vi "JSON to Array of Cluster.vi"(5 "JSON":string, 6 "JSONtext LVClass Serializer in":refnum<class "JSONtext LVClass Serializer.lvclass">, 7 "Item Offset":i32[](array[numeric]), 8 "error in (no error)":errorcluster, 9 "Element Info":T3(array[cluster]), 10 "Elements":variant[](array[variant]), 11 "ELement Names":string[](array[string])) -> (0 "error out":errorcluster, 3 "Cluster of Variants":variant[](array[variant]))   [LabVIEW 2024, in "JSONtext.lvlib"]
uses:
  JSONtext.lvlib
  JSONtext LVClass Serializer.lvclass
  Data Type.ctl
  Tag Type.ctl
  NI_Data Type.lvlib
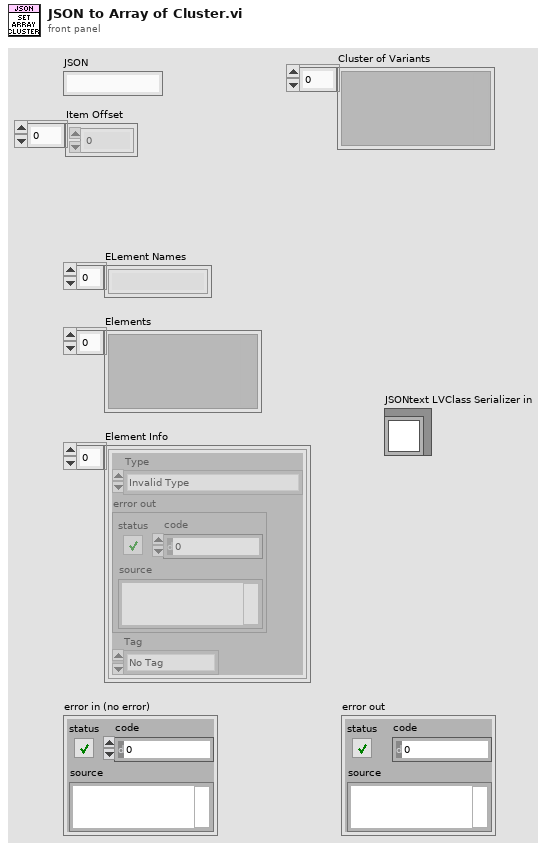
[diagram p1: front panel]
types:
  T1 = typedef "NI_Data Type.lvlib/Data Type.ctl" = enum8{"Invalid Type", "Void", "I8", "I16", "I32", "I64", "U8", "U16", "U32", "U64", "Single Float", "Double Float", "Extended Float", "Single Complex", "Double Complex", "Extended Complex", "Enum U8", "Enum U16", "Enum U32", "Enum U64", "Single Float With Unit", "Double Float With Unit", "Extended Float With Unit", "Single Complex with Unit", "Double Complex with Unit", "Extended Complex with Unit", "Boolean", "String", "Path", "Picture", "Tag", "Array", "Cluster", "Variant", "LV Variant", "Waveform", "Timestamp", "Digital Waveform", "Digital Data", "ExpressData", "Refnum", "External Data", "VI", "Poly VI", "LabVIEW Class Instance", "Fixed Point", "Set Collection", "Map Collection"}
  T2 = typedef "JSONtext.lvlib/Tag Type.ctl" = enum16{"No Tag", "<JSON>", "<JOBJ>", "<UTF8>"}
  T3 = cluster{"Type":T1, "error out":errorcluster, "Tag":T2}[]
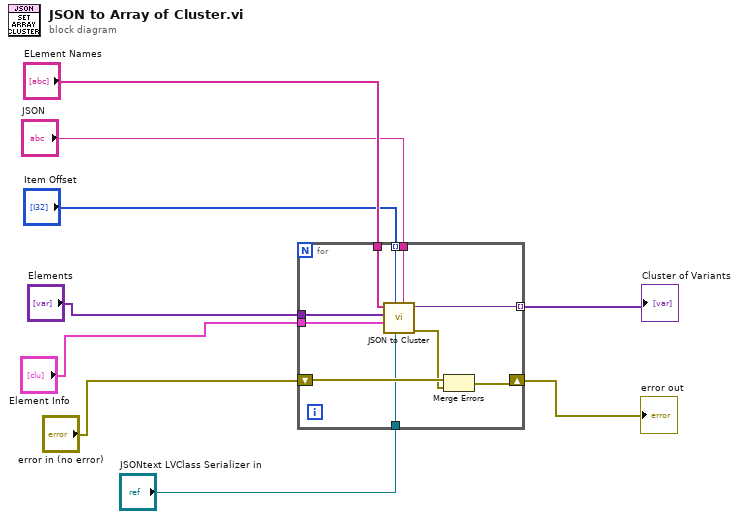
[diagram p0: block diagram]
diagram:
  n1 = for {
    tunnel: "ELement Names" -> [w19]
    tunnel: "JSON" -> [w18]
    tunnel: "Item Offset" -> [w17] mode=indexing
    tunnel: "Elements" -> [w16]
    tunnel: "Element Info" -> [w15]
    shift-right: [w12] -> w2
    shift-left: "error in (no error)" -> [w14]
    tunnel: [w11] -> w3 mode=indexing
    tunnel: "JSONtext LVClass Serializer in" -> [w10]
    n2 = call "JSON to Cluster.vi"("JSON"=w18, "JSONtext LVClass Serializer in"=w10, "Item Offset"=w17, "Element Info"=w15, "Elements"=w16, "ELement Names (as JSON)"=w19) -> ("error out"=w13:errorcluster, "Cluster of Variants"=w11:variant)  [unwired: 4 in]
    n3 = Merge Errors(w14, w13) -> (w12:errorcluster)
  }
  "Cluster of Variants" <- w3
  "error out" <- w2
